vi "Try 1.vi"() -> ()   [LabVIEW 2014]
uses:
  <vilib>/Aledyne-TSXperts/Arduino Compatible Compiler for LabVIEW/addons/Arduino TFT/Arduino TFT.lvlib
panel:
  out "Error Out":errorcluster
  in  "Error In":errorcluster
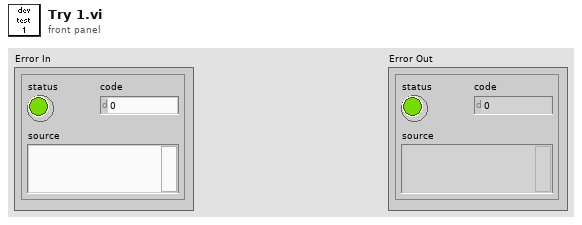
[diagram p1: front panel]
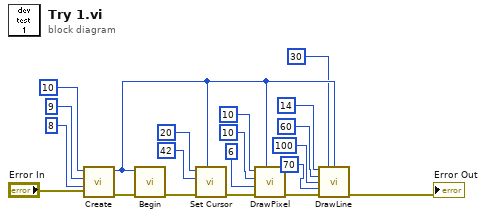
[diagram p0: block diagram]
diagram:
  n1 = call <vilib>:"Create.vi"("Error In"="Error In", "rst"=u8 8 ("cs"), "rs"=u8 9 ("cs"), "cs"=u8 10) -> ("Error Out"=w19:errorcluster, "Instance"=w11:u32)  [unwired: 4 in]
  n2 = call <vilib>:"Begin.vi"("Error In"=w19, "Instance"=w11) -> ("Error Out"=w18:errorcluster)  [unwired: 8 in]
  n3 = call <vilib>:"Set Cursor.vi"("Instance"=w11, "Error In"=w18, "y"=i16 42 ("x"), "x"=i16 20) -> ("Error Out"=w17:errorcluster)  [unwired: 7 in]
  n4 = call <vilib>:"DrawPixel.vi"("Instance"=w11, "Error In"=w17, "color"=u8 6 ("x"), "y"=u8 10 ("x"), "x"=u8 10) -> ("Error Out"=w16:errorcluster)  [unwired: 6 in]
  n5 = call <vilib>:"DrawLine.vi"("x"=i16 14, "color"=u8 30, "Instance"=w11, "y"=i16 60 ("x"), "x2"=i16 100 ("x"), "y2"=i16 70 ("x"), "Error In"=w16) -> ("Error Out"=→"Error Out":errorcluster)  [unwired: 8 in]
